vi "Is_it_a_Results_File.vi"(0 "character string":string) -> (1 "Contain DB Header Info":bool, 2 "Header String":string, 3 "Results File?":bool)   [LabVIEW 2012]
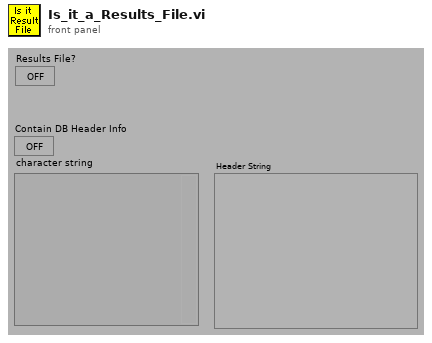
[diagram p1: front panel]
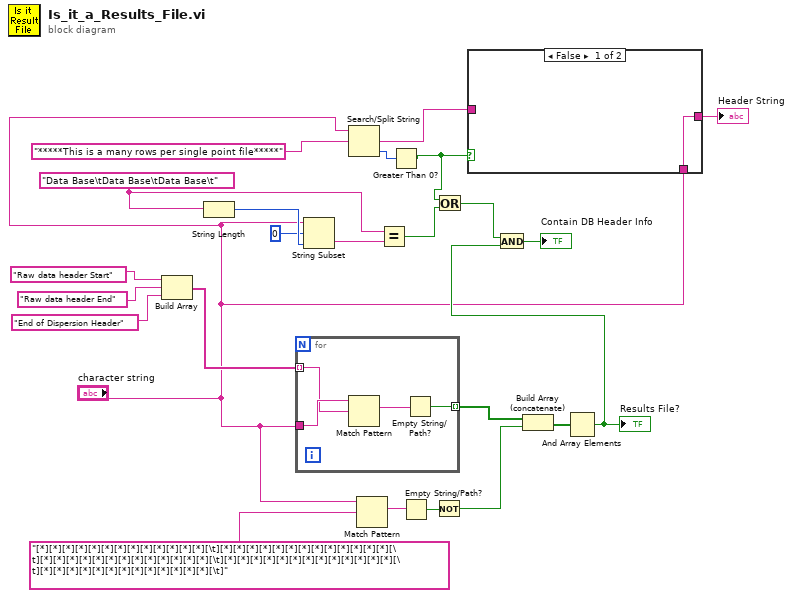
[diagram p0: block diagram]
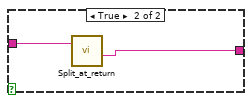
[diagram p2: hidden frame]
diagram:
  w11 = "Data Base\tData Base\tData Base\t"
  n1 = Build Array("Raw data header Start", "Raw data header End", "End of Dispersion Header") -> (w22:string[])
  n2 = String Length(string=w11) -> (length=w14:i32)
  n3 = for {
    tunnel: "character string" -> [w28]
    tunnel: w22 -> [w27] mode=indexing
    tunnel: [w25] -> w19 mode=indexing
    n4 = Match Pattern(string=w28, regular expression=w27) -> (match substring=w26:string)  [unwired: 4 out]
    n5 = Empty String/Path?(string/path=w26) -> (empty?=w25:bool)
  }
  n6 = String Subset(string="character string", offset (0)=0, length (rest)=w14) -> (substring=w12:string)
  n7 = Search/Split String(string="character string", search string/char (-)="*****This is a many rows per single point file*****") -> (match + rest of string=w6:string, offset of match=w2:i32)  [unwired: 2 out]
  n8 = Match Pattern(string="character string", regular expression="[*][*][*][*][*][*][*][*][*][*][*][*][*][\t][*][*][*][*][*][*][*][*][*][*][*][*][*][\t][*][*][*][*][*][*][*][*][*][*][*][*][*][\t][*][*][*][*][*][*][*][*][*][*][*][*][*][\t][*][*][*][*][*][*][*][*][*][*][*][*][*][\t]" ("String")) -> (match substring=w21:string)  [unwired: 4 out]
  n9 = Equal?(x=w11, y=w12) -> (x = y?=w8:bool)
  n10 = Greater Than 0?(x=w2) -> (x > 0?=w1:bool)
  n11 = Empty String/Path?(string/path=w21) -> (empty?=w20:bool)
  n12 = Not(x=w20) -> (.not. x?=w18:bool)
  n13 = Or(x=w1, y=w8) -> (x .or. y?=w7:bool)
  n14 = case shown="False" w1 {
    tunnel: w6 -> [_ w31]
    tunnel: [w29 w30] -> w5
    tunnel: "character string" -> [w29 _]
    frame False {
    }
    frame True {
      n15 = call "Split_at_return.vi"("String"=w31) -> ("after substring"=w30:string)  [unwired: 1 in, 3 out]
    }
  }
  "Header String" <- w5
  n16 = Build Array (concatenate)(w19, w18) -> (w17:bool[])
  n17 = And Array Elements(Boolean array=w17) -> (logical AND=w10:bool)
  "Results File?" <- w10
  n18 = And(x=w7, y=w10) -> (x .and. y?=→"Contain DB Header Info":bool)
